vi "V2H_L.vi"(2 "YL in":dbl[](array[numeric]), 3 "XL in":dbl[](array[numeric])) -> (0 "YL out":dbl[](array[numeric]), 1 "XL out":dbl[](array[numeric]))   [LabVIEW 2014]
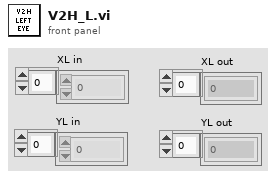
[diagram p1: front panel]
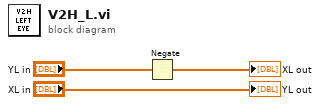
[diagram p0: block diagram]
diagram:
  n1 = Negate(x="YL in") -> (-x=→"XL out":dbl[])
  "YL out" <- "XL in"
